vi "Initialize.vi"(8 "error in (no error)":errorcluster) -> (0 "error out":errorcluster)   [LabVIEW 2019, in "Camera Engine.lvlib"]
uses:
  Camera Engine.lvlib
  Global.vi
panel:
  # "Input"
  # "Output"
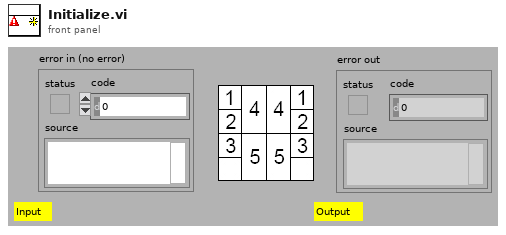
[diagram p1: front panel]
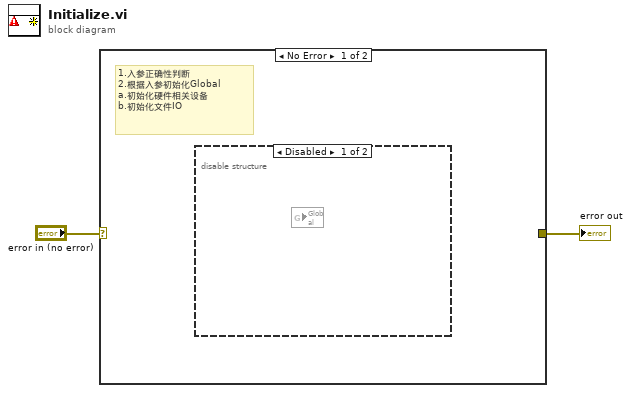
[diagram p0: block diagram]
diagram:
  n1 = case shown="No Error" "error in (no error)" {
    selector: "error in (no error)" -> [_ w3]
    tunnel: [_ w3] -> w1
    frame No Error {
      # "1.入参正确性判断\n2.根据入参初始化Global\na.初始化硬件相关设备\nb.初始化文件IO"
      n2 = disable-structure shown="Disabled" {
        frame Disabled {
          n3 = global read "Global.vi" item#-1() -> ()  [unwired: 1 in]
        }
        frame Enabled {
        }
      }
    }
    frame Error {
    }
  }
  "error out" <- w1
